vi "WBRT Controller.vi"(4 "Loop count":i32, 6 "Elapsed Time":dbl, 7 "Manual Motor Control":bool, 8 "error in (no error)":errorcluster, 11 "WBRT State In":T2={"Encoders"={"Roll"=0.0, "Pitch"=0.0, "Yaw"=0.0, "Roll Trim"=0.0, "Pitch Trim"=0.0, "Yaw Trim"=0.0, "Roll Rate"=0.0, "Pitch Rate"=0.0, "Yaw Rate"=0.0}, "SPI Data"={"X-Gyro"=0.0, "Y-Gyro"=0.0, "Z-Gyro"=0.0, "X-Accel"=0.0, "Y-Accel"=0.0, "Z-Accel"=0.0}, "Camera"={"Numeric"=0.0}, "Filter Data"={"Filter Enabled?"=FALSE, "Filter Type"=enum."Equi-Ripple", "Pass Frequency"=1.0, "Stop Frequency (Equi-Ripple)"=0.45000000000000007, "Order"=0, "Ripple (dB)"=2.0}, "FPGA VI Reference"=refnum, "dt"=0.0, "Elapsed Time (msec)"=0, "Setpoints"={"Roll Setpoint (degrees)"=125.0, "Pitch Setpoint (degrees)"=125.0, "Yaw Setpoint (degrees)"=125.0}, "Commands"={"Left Command"=0.0, "Right Command"=0.0}, "Trajectory Data"=[], "Gains"={"Gain1"=0.0, "Gain2"=0.0, "Gain3"=0.0, "Gain4"=0.0, "Gain5"=0.0, "Gain6"=0.0, "Gain7"=0.0, "Gain8"=0.0, "Gain9"=0.0}, "Global Variables"={"Variable1"=[], "Variable2"=[], "Variable3"=[], "Variable4"=[]}, "Centroid"={"X Centroid"=0.0, "Y Centroid"=0.0}, "Error1"=0.0, "Error2"=0.0, "Error3"=0.0, "Error4"=0.0, "Recorded Data"=[], "Landing Factor"=0.0} {"Trajectory Data" format="%0.3f"; "Filter Data"."Stop Frequency (Equi-Ripple)" format="%0.3f"; "Filter Data"."Pass Frequency" format="%0.3f"}) -> (0 "error out":errorcluster, 3 "WBRT State Out":T2={"Encoders"={"Roll"=0.0, "Pitch"=0.0, "Yaw"=0.0, "Roll Trim"=0.0, "Pitch Trim"=0.0, "Yaw Trim"=0.0, "Roll Rate"=0.0, "Pitch Rate"=0.0, "Yaw Rate"=0.0}, "SPI Data"={"X-Gyro"=0.0, "Y-Gyro"=0.0, "Z-Gyro"=0.0, "X-Accel"=0.0, "Y-Accel"=0.0, "Z-Accel"=0.0}, "Camera"={"Numeric"=0.0}, "Filter Data"={"Filter Enabled?"=FALSE, "Filter Type"=enum."Equi-Ripple", "Pass Frequency"=1.0, "Stop Frequency (Equi-Ripple)"=0.45000000000000007, "Order"=0, "Ripple (dB)"=2.0}, "FPGA VI Reference"=refnum, "dt"=0.0, "Elapsed Time (msec)"=0, "Setpoints"={"Roll Setpoint (degrees)"=125.0, "Pitch Setpoint (degrees)"=125.0, "Yaw Setpoint (degrees)"=125.0}, "Commands"={"Left Command"=0.0, "Right Command"=0.0}, "Trajectory Data"=[], "Gains"={"Gain1"=0.0, "Gain2"=0.0, "Gain3"=0.0, "Gain4"=0.0, "Gain5"=0.0, "Gain6"=0.0, "Gain7"=0.0, "Gain8"=0.0, "Gain9"=0.0}, "Global Variables"={"Variable1"=[], "Variable2"=[], "Variable3"=[], "Variable4"=[]}, "Centroid"={"X Centroid"=0.0, "Y Centroid"=0.0}, "Error1"=0.0, "Error2"=0.0, "Error3"=0.0, "Error4"=0.0, "Recorded Data"=[], "Landing Factor"=0.0} {"Trajectory Data" format="%0.3f"; "Filter Data"."Stop Frequency (Equi-Ripple)" format="%0.3f"; "Filter Data"."Pass Frequency" format="%0.3f"}, 5 "Error Chart Cluster":T1)   [LabVIEW 2012]
doc: "This VI contains a mathscript node where a user must define a controller for the Whirlybird. All inputs are defined on the left edge of the mathscript node and the outputs are defined on the right. Users can still define other variables within the mathscript node.\n\nAuthor: Brandon Steele\n\nCopyright: Brigham Young University"
uses:
  Supporting Files/Custom Controls/WBRT State.ctl
  Supporting Files/Custom Controls/WBRT Encoders.ctl
  Supporting Files/Custom Controls/WBRT SPI Data.ctl
  Supporting Files/Custom Controls/WBRT Filter Data.ctl
  Supporting Files/Custom Controls/WBRT Filter Type.ctl
  Supporting Files/FPGA Samples/spi_single port_example/Host API/Controls/FPGA SPI_FPGA Ref.ctl
  Supporting Files/Custom Controls/WBRT Setpoints.ctl
  Supporting Files/Custom Controls/WBRT Commands.ctl
  Supporting Files/Custom Controls/WBRT Gains.ctl
  Supporting Files/Custom Controls/WBRT Global Variables.ctl
  <vilib>/imath/engines/lvmath2/RunTimeEngine/ErrorHandling/NIMS_Finalize Error.vi
  <vilib>/imath/engines/lvmath2/RunTimeEngine/NodeEndStatement/NIMS_NodeEndStatement_Output.vi
  <instcachedir>/0/NIMS_NodeEndStatement_Output_53EC0D466D134D7ABD903AC30B43404B.lvgen/NIMS_NodeEndStatement_Output_53EC0D466D134D7ABD903AC30B43404B_001.vi
  <instcachedir>/0/NIMS_NodeEndStatement_Output_53EC0D466D134D7ABD903AC30B43404B.lvgen/NIMS_NodeEndStatement_Output_53EC0D466D134D7ABD903AC30B43404B_002.vi
  <vilib>/imath/engines/lvmath2/RunTimeEngine/ReplaceToken/NIMS_Replace - Check Linear.vi
  <instcachedir>/0/NIMS_Replace - Check Linear_44ABB4D6A819426DBDF25CCE6827BF1D.lvgen/NIMS_Replace - Check Linear_44ABB4D6A819426DBDF25CCE6827BF1D_010.vi
  <vilib>/imath/engines/lvmath2/RunTimeEngine/ReplaceToken/NIMS_Replace - Size Check _(_)=S.vi
  <instcachedir>/0/NIMS_Replace - Size Check _(_)=S_5AC8AA27B9694BB9828B57BCF666F597.lvgen/NIMS_Replace - Size Check _(_)=S_5AC8AA27B9694BB9828B57BCF666F597_006.vi
  <vilib>/imath/engines/lvmath2/RunTimeEngine/ReplaceToken/NIMS_Replace - M(S)=S.vi
  <instcachedir>/0/NIMS_Replace - M(S)=S_44490A2B072F4ABCB49D645629E85292.lvgen/NIMS_Replace - M(S)=S_44490A2B072F4ABCB49D645629E85292_000.vi
  <vilib>/imathl/engines/lvmath/Functions/Error Handling/Create Error.vi
  <vilib>/imath/engines/lvmath2/RunTimeEngine/VariableToken/Read/NIMS_Get Elements - SorM(_) - Check.vi
  <instcachedir>/0/NIMS_Get Elements - SorM(_) - Check_8FDA2664A675493882C25203DD903B51.lvgen/NIMS_Get Elements - SorM(_) - Check_8FDA2664A675493882C25203DD903B51_000.vi
  <vilib>/imath/engines/lvmath2/RunTimeEngine/BuiltInFunctions/abs/NIMS_abs(signed).vi
  <instcachedir>/0/NIMS_abs(signed)_C4FCB8E6058B49B797C7C8D53CA5F6EC.lvgen/NIMS_abs(signed)_C4FCB8E6058B49B797C7C8D53CA5F6EC_000.vi
panel:
  # "Press Control + E to open block diagram\nor\nClick Window -> Show Block Diagram"
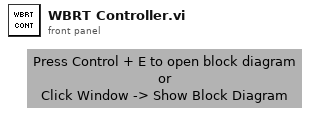
[diagram p1: front panel]
types:
  T1 = cluster{"[0]":dbl, "[1]":dbl, "[2]":dbl, "[3]":dbl}
  T2 = typedef "WBRT State.ctl" = cluster{"Encoders":T3, "SPI Data":T4, "Camera":cluster{"Numeric":dbl}, "Filter Data":T5, "FPGA VI Reference":T7, "dt":dbl, "Elapsed Time (msec)":u32, "Setpoints":T8, "Commands":T9, "Trajectory Data":dbl[][], "Gains":T10, "Global Variables":T11, "Centroid":cluster{"X Centroid":sgl, "Y Centroid":sgl}, "Error1":dbl, "Error2":dbl, "Error3":dbl, "Error4":dbl, "Recorded Data":dbl[][], "Landing Factor":dbl}
  T3 = typedef "WBRT Encoders.ctl" = cluster{"Roll":dbl, "Pitch":dbl, "Yaw":dbl, "Roll Trim":dbl, "Pitch Trim":dbl, "Yaw Trim":dbl, "Roll Rate":dbl, "Pitch Rate":dbl, "Yaw Rate":dbl}
  T4 = typedef "WBRT SPI Data.ctl" = cluster{"X-Gyro":dbl, "Y-Gyro":dbl, "Z-Gyro":dbl, "X-Accel":dbl, "Y-Accel":dbl, "Z-Accel":dbl}
  T5 = typedef "WBRT Filter Data.ctl" = cluster{"Filter Enabled?":bool, "Filter Type":T6, "Pass Frequency":dbl, "Stop Frequency (Equi-Ripple)":dbl, "Order":i32, "Ripple (dB)":dbl}
  T6 = typedef "WBRT Filter Type.ctl" = enum16{"Equi-Ripple", "Butterworth", "Chebyshev"}
  T7 = typedef "FPGA SPI_FPGA Ref.ctl" = refnum<k20>
  T8 = typedef "WBRT Setpoints.ctl" = cluster{"Roll Setpoint (degrees)":dbl, "Pitch Setpoint (degrees)":dbl, "Yaw Setpoint (degrees)":dbl}
  T9 = typedef "WBRT Commands.ctl" = cluster{"Left Command":dbl, "Right Command":dbl}
  T10 = typedef "WBRT Gains.ctl" = cluster{"Gain1":dbl, "Gain2":dbl, "Gain3":dbl, "Gain4":dbl, "Gain5":dbl, "Gain6":dbl, "Gain7":dbl, "Gain8":dbl, "Gain9":dbl}
  T11 = typedef "WBRT Global Variables.ctl" = cluster{"Variable1":dbl[][], "Variable2":dbl[][], "Variable3":dbl[][], "Variable4":dbl[][]}
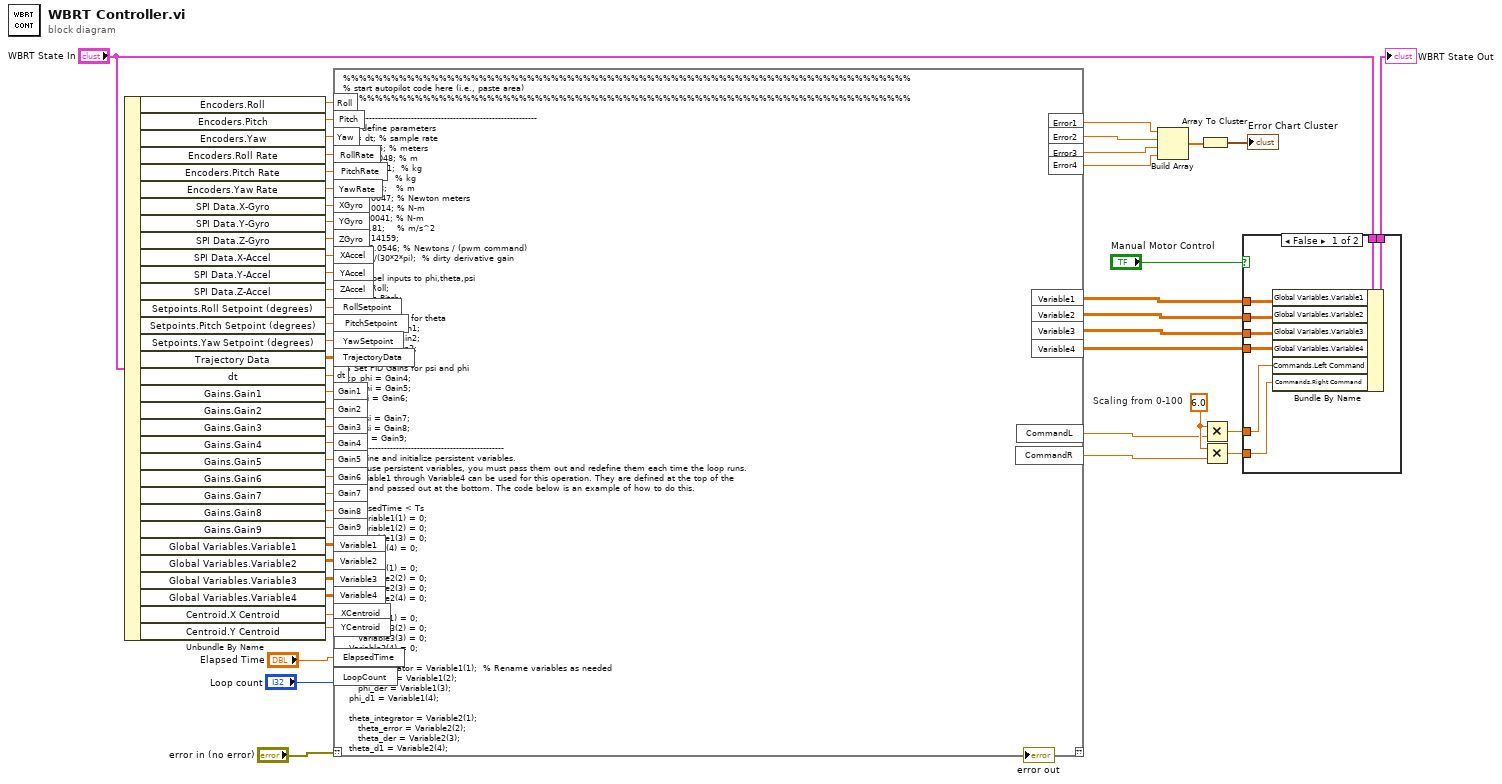
[diagram p0: block diagram]
diagram:
  w23 = 6.0  # Scaling from 0-100
  n1 = Unbundle By Name("WBRT State In") -> ("Encoders.Roll"=w54:dbl, "Encoders.Pitch"=w53:dbl, "Encoders.Yaw"=w52:dbl, "Encoders.Roll Rate"=w36:dbl, "Encoders.Pitch Rate"=w35:dbl, "Encoders.Yaw Rate"=w34:dbl, "SPI Data.X-Gyro"=w37:dbl, "SPI Data.Y-Gyro"=w51:dbl, "SPI Data.Z-Gyro"=w50:dbl, "SPI Data.X-Accel"=w49:dbl, "SPI Data.Y-Accel"=w48:dbl, "SPI Data.Z-Accel"=w47:dbl, "Setpoints.Roll Setpoint (degrees)"=w42:dbl, "Setpoints.Pitch Setpoint (degrees)"=w41:dbl, "Setpoints.Yaw Setpoint (degrees)"=w40:dbl, "Trajectory Data"=w38:dbl[][], "dt"=w39:dbl, "Gains.Gain1"=w32:dbl, "Gains.Gain2"=w31:dbl, "Gains.Gain3"=w30:dbl, "Gains.Gain4"=w29:dbl, "Gains.Gain5"=w28:dbl, "Gains.Gain6"=w27:dbl, "Gains.Gain7"=w26:dbl, "Gains.Gain8"=w25:dbl, "Gains.Gain9"=w24:dbl, "Global Variables.Variable1"=w22:dbl[][], "Global Variables.Variable2"=w21:dbl[][], "Global Variables.Variable3"=w20:dbl[][], "Global Variables.Variable4"=w19:dbl[][], "Centroid.X Centroid"=w12:sgl, "Centroid.Y Centroid"=w11:sgl)
  n2 = mathscript code="%%%%%%%%%%%%%%%%%%%%%%%%%%%%%%%%%%%%%%%%%%%%%%%%%%%%%%%%%%%%%%%%%%%%%%%\n% start autopilot code here (i.e., paste area)\n%%%%%%%%%%%%%%%%%%%%%%%%%%%%%%%%%%%%%%%%%%%%%%%%%%%%%%%%%%%%%%%%%%%%%%%\n\n%--------------------------------------------------------------\n%% define parameters\nTs = dt; % sample rate\nL1 = 0.85; % meters\nL2 = 0.3048; % m\nm1 = 0.891;  % kg\nm2 = 1;      % kg\nd = 0.178;   % m\nJx = 0.0047; % Newton meters\nJy = 0.0014; % N-m\nJz = 0.0041; % N-m\ng  = 9.81;    % m/s^2\npi = 3.14159;\nkm = 0.0546; % Newtons / (pwm command)\ntau = 1/(30*2*pi);  % dirty derivative gain\n\n% Relabel inputs to phi,theta,psi\n\tphi = Roll;\n\ttheta = Pitch;\n\tpsi = Yaw;\n% Set PID Gains for theta\n\tkp_theta = Gain1;\n\tkd_theta = Gain2;\n\tki_theta = Gain3;\n\t\n% Set PID Gains for psi and phi\n\tkp_phi = Gain4;\n\tkd_phi = Gain5;\n\tki_phi = Gain6;\n\t\n\tkp_psi = Gain7;\n\tkd_psi = Gain8;\n\tki_psi = Gain9;\n%---------------------------------------------------\n% define and initialize persistent variables.\n% To use persistent variables, you must pass them out and redefine them each time the loop runs. \n% Variable1 through Variable4 can be used for this operation. They are defined at the top of the \n% file and passed out at the bottom. The code below is an example of how to do this.\n\nif ElapsedTime < Ts\n     Variable1(1) = 0;\n     Variable1(2) = 0;\n     Variable1(3) = 0;\n\t Variable1(4) = 0;\t \n\t \n\t Variable2(1) = 0;\n     Variable2(2) = 0;\n     Variable2(3) = 0;\n     Variable2(4) = 0;\t \n\t \n\t Variable3(1) = 0;\n     Variable3(2) = 0;\n     Variable3(3) = 0;\n\t Variable3(4) = 0;\t \nend\n     phi_integrator = Variable1(1);  % Rename variables as needed\n     phi_error = Variable1(2);\n     phi_der = Variable1(3);\n\t phi_d1 = Variable1(4);\n\t \n\t theta_integrator = Variable2(1);\n     theta_error = Variable2(2);\n     theta_der = Variable2(3);\n\t theta_d1 = Variable2(4);\n\t \n\t psi_der = Variable3(1);\n     psi_error = Variable3(2);\n     psi_d1 = Variable3(3);\n\t psi_intergrator = Variable3(4);\n\n\n%---------------------------------------------------\n% convert PitchSetpoint and YawSetpoint to radians\nPitchSetpoint = PitchSetpoint *(pi/180);\nYawSetpoint = YawSetpoint * (pi/180);\n\nFe = g*(m1*L1 - m2*L2)/L1;\nF_max = 10.92;\n\n%---------------------------------------------------\n% longitudinal controller\n\n% feedforward pitch command\nF_ff = Fe*cos(PitchSetpoint);\n\t\n% PID PITCH LOOP \nerror1 = PitchSetpoint - theta;\n\ntheta_integrator = theta_integrator  + (Ts/2) * (error1 + theta_error);\n\ntheta_der = (2*tau-Ts)/(2*tau+Ts)*theta_der + 2/(2*tau+Ts)*(theta - theta_d1);\n\ntheta_error = error1;\n\ntheta_d1 = theta;\n\nun_saturation = kp_theta*error1 +ki_theta*theta_integrator - kd_theta * theta_der + F_ff;\n\nif (un_saturation > F_max)\n\tF_tilde = F_max;\nelseif (un_saturation< - F_max)\n\tF_tilde = -F_max;\nelse\n\tF_tilde = un_saturation;\nend\n\nF = Fe + F_tilde;\n%---------------------------------------------------\n%lateral controller\n\t\n% PID YAW LOOP \nerror2 = YawSetpoint - psi;\npsi_der = (2*tau-Ts)/(2*tau+Ts)*psi_der + 2/(2*tau+Ts)*(psi-psi_d1);\nif abs(psi_error)>15*pi/180\n      psi_intergrator = 0;\nelse\n     psi_intergrator = psi_intergrator + (Ts/2)*(error2+psi_error);\nend\npsi_error = error2;\npsi_d1 = psi;\n\nun_saturation2 = kp_psi*error2 + ki_psi*psi_intergrator - kd_psi*psi_der;\nRollSetpoint = un_saturation2;\n\n% PID ROLL LOOP \nerror3 = RollSetpoint - phi;\nif abs(phi_error)>15*pi/180\n      phi_intergrator = 0;\nelse\n     phi_integrator = phi_integrator + (Ts/2)*(error3+phi_error);\nend\nphi_der = (2* tau-Ts)/ (2 * tau + Ts) * phi_der + 2/(2*tau+Ts)*(phi - phi_d1);\nphi_error = error3;\nphi_d1 = phi;\n\nTau_tilde = kp_phi*error3+ ki_phi * phi_integrator - kd_phi*phi_der;\n\n%---------------------------------------------------\n% update persistent variables\n\n% done throughout the code\n\n%---------------------------------------------------\n% Pass Persistent Variables Out\n% Rename variables as needed\nVariable1 = [phi_integrator; phi_error; phi_der; phi_d1;]; % This vector can be of any length.\nVariable2 = [theta_integrator; theta_error; theta_der; theta_d1];\nVariable3 = [psi_der; psi_error; psi_d1; psi_intergrator];\n\n\n%%%%%%%%%%%%%%%%%%%%%%%%%%%%%%%%%%%%%%%%%%%%%%%%%%%%%%%%%%%%%%%%%%%%%%%\n% stop autopilot code here (i.e., paste area)\n%%%%%%%%%%%%%%%%%%%%%%%%%%%%%%%%%%%%%%%%%%%%%%%%%%%%%%%%%%%%%%%%%%%%%%%  \n\n\n%---------------------------------------------------------------\n% Convert force and torque to PWM outputs (don't change this)\n  CommandL  = 1/2/km*(F + Tau_tilde/d);\n  CommandR = 1/2/km*(F - Tau_tilde/d);\n  \n  % saturate PWM signals\n  if CommandL > 100, CommandL=100;\n  elseif CommandL < 0, CommandL = 0;\n  end\n  if CommandR > 100, CommandR=100;\n  elseif CommandR < 0, CommandR = 0;\n  end\n\n  pwm_commands = [CommandL; CommandR];\n  \nError1=LoopCount;\nError2=ElapsedTime;\nError3=0;\nError4=0;"("??"="error in (no error)", "Roll"=w54, "Pitch"=w53, "Yaw"=w52, "XGyro"=w37, "YGyro"=w51, "ZGyro"=w50, "XAccel"=w49, "YAccel"=w48, "ZAccel"=w47, "RollSetpoint"=w42, "PitchSetpoint"=w41, "YawSetpoint"=w40, "dt"=w39, "TrajectoryData"=w38, "RollRate"=w36, "PitchRate"=w35, "YawRate"=w34, "Gain1"=w32, "Gain2"=w31, "Gain3"=w30, "Gain4"=w29, "Gain5"=w28, "Gain6"=w27, "Gain7"=w26, "Gain8"=w25, "Gain9"=w24, "Variable1"=w22, "Variable2"=w21, "Variable3"=w20, "Variable4"=w19, "XCentroid"=w12, "YCentroid"=w11, "ElapsedTime"="Elapsed Time", "LoopCount"="Loop count") -> ("??"=→"error out":errorcluster, "CommandL"=w5:dbl, "CommandR"=w4:dbl, "Variable1"=w18:dbl[][], "Variable2"=w17:dbl[][], "Variable3"=w16:dbl[][], "Variable4"=w15:dbl[][], "Error1"=w10:dbl, "Error2"=w9:dbl, "Error3"=w8:dbl, "Error4"=w7:dbl)
  n3 = Build Array(w10, w9, w8, w7) -> (w6:dbl[])
  n4 = Array To Cluster(array=w6) -> (cluster=→"Error Chart Cluster":T1)
  n5 = Multiply(x=w23, y=w5) -> (x*y=w14:dbl)
  n6 = Multiply(x=w23, y=w4) -> (x*y=w13:dbl)
  n7 = case shown="False" "Manual Motor Control" {
    tunnel: "WBRT State In" -> [w62 w63]
    tunnel: [w61 w63] -> w45
    tunnel: w18 -> [w60 _]
    tunnel: w17 -> [w59 _]
    tunnel: w16 -> [w58 _]
    tunnel: w15 -> [w57 _]
    tunnel: w14 -> [w55 _]
    tunnel: w13 -> [w56 _]
    frame False {
      n8 = Bundle By Name(cluster=w62, "Global Variables.Variable1"=w60, "Global Variables.Variable2"=w59, "Global Variables.Variable3"=w58, "Global Variables.Variable4"=w57, "Commands.Left Command"=w55, "Commands.Right Command"=w56) -> (w61:T2)
    }
    frame True {
    }
  }
  "WBRT State Out" <- w45
